vi "myRIO_BRig_RT__MTrig_increment.vi"(0 "input_dataMTrig":u16[](array[numeric]), 2 "input_Solenoid__L":bool, 3 "input_Solenoid__R":bool, 4 "input_Audio__L":bool, 5 "input_Audio__R":bool, 9 "input_Laser":bool) -> (14 "output_dataMTrig":u16[](array[numeric]))   [LabVIEW 2014]
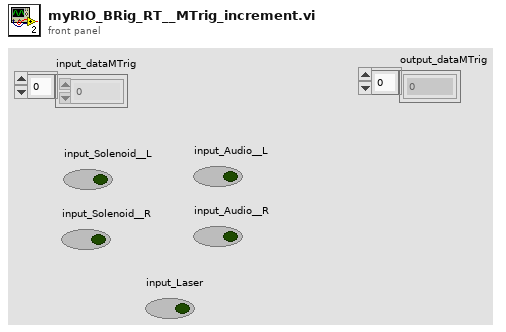
[diagram p1: front panel]
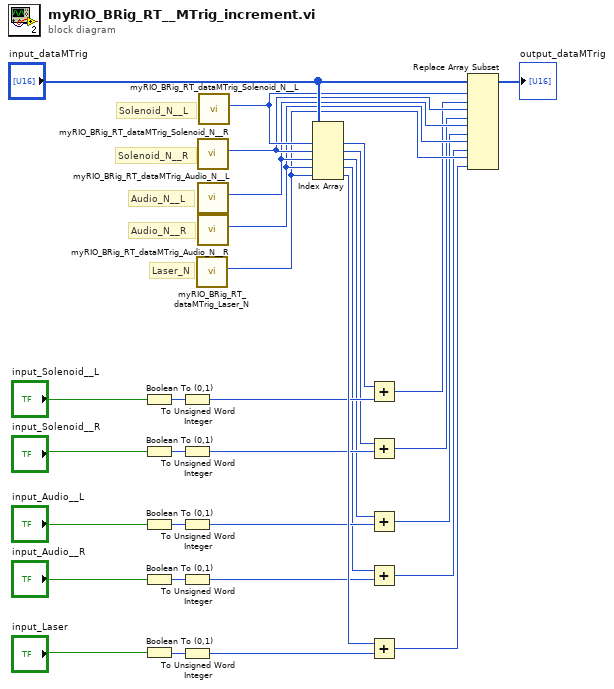
[diagram p0: block diagram]
diagram:
  # "Laser_N"
  # "Audio_N__R"
  # "Audio_N__L"
  # "Solenoid_N__R"
  # "Solenoid_N__L"
  n1 = Boolean To (0,1)(Boolean="input_Solenoid__L") -> (0, 1=w11:i16)
  n2 = Boolean To (0,1)(Boolean="input_Solenoid__R") -> (0, 1=w13:i16)
  n3 = Boolean To (0,1)(Boolean="input_Audio__L") -> (0, 1=w15:i16)
  n4 = Boolean To (0,1)(Boolean="input_Audio__R") -> (0, 1=w17:i16)
  n5 = Boolean To (0,1)(Boolean="input_Laser") -> (0, 1=w19:i16)
  n6 = To Unsigned Word Integer(number=w11) -> (unsigned 16bit integer=w10:u16)
  n7 = To Unsigned Word Integer(number=w13) -> (unsigned 16bit integer=w12:u16)
  n8 = To Unsigned Word Integer(number=w15) -> (unsigned 16bit integer=w14:u16)
  n9 = To Unsigned Word Integer(number=w17) -> (unsigned 16bit integer=w16:u16)
  n10 = To Unsigned Word Integer(number=w19) -> (unsigned 16bit integer=w18:u16)
  n11 = call "myRIO_BRig_RT_dataMTrig_Laser_N.vi"() -> ("output_Laser_c"=w26:i32)  [unwired: 11 in]
  n12 = call "myRIO_BRig_RT_dataMTrig_Solenoid_N__R.vi"() -> ("output_Solenoid_N__R"=w29:i32)  [unwired: 11 in]
  n13 = call "myRIO_BRig_RT_dataMTrig_Audio_N__L.vi"() -> ("output_Audio_N__L"=w28:i32)  [unwired: 11 in]
  n14 = call "myRIO_BRig_RT_dataMTrig_Audio_N__R.vi"() -> ("output_Audio_N__R"=w27:i32)  [unwired: 11 in]
  n15 = call "myRIO_BRig_RT_dataMTrig_Solenoid_N__L.vi"() -> ("output_Solenoid_N__L"=w30:i32)  [unwired: 11 in]
  n16 = Index Array(array="input_dataMTrig", index #1=w30, index #2=w29, index #3=w28, index #4=w27, index #5=w26) -> (element #1=w6:u16, element #2=w7:u16, element #3=w8:u16, element #4=w9:u16, element #5=w20:u16)
  n17 = Add(x=w6, y=w10) -> (x+y=w5:u16)
  n18 = Add(x=w7, y=w12) -> (x+y=w4:u16)
  n19 = Add(x=w8, y=w14) -> (x+y=w3:u16)
  n20 = Add(x=w9, y=w16) -> (x+y=w2:u16)
  n21 = Add(x=w20, y=w18) -> (x+y=w1:u16)
  n22 = Replace Array Subset(array="input_dataMTrig", new element #1=w5, index #1=w30, new element #2=w4, index #2=w29, new element #3=w3, index #3=w28, new element #4=w2, index #4=w27, new element #5=w1, index #5=w26) -> (→"output_dataMTrig":u16[])
